vi "Complete Call.vi"(0 "gRPCid":T1, 3 "error in":errorcluster) -> (10 "error out":errorcluster)   [LabVIEW 2019, in "grpc-lvsupport.lvlib"]
uses:
  grpc-lvsupport.lvlib
  grpcId.ctl
  <vilib>/Utility/error.llb/Error Cluster From Error Code.vi
  <resource>/libgrpc_labview.dll
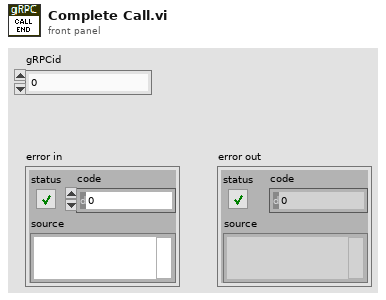
[diagram p1: front panel]
types:
  T1 = typedef "grpc-lvsupport.lvlib/grpcId.ctl" = u64
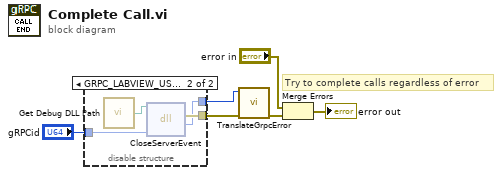
[diagram p0: block diagram]
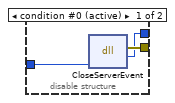
[diagram p2: hidden frame]
diagram:
  # "Try to complete calls regardless of error"
  n1 = disable-structure shown="GRPC_LABVIEW_USE_DEBUG_DLL==True&&RUN_TIME_ENGINE==False" {
    disable-tunnel: [w9 w13] -> w6
    disable-tunnel: "gRPCid" -> [w8 w12]
    disable-tunnel: [w7 w10] -> w3
    frame condition #0 (active) {
      n2 = dll-call lib="C:/Program Files (x86)/National Instruments/LabVIEW 2024/resource/libgrpc_labview.*" fn="CloseServerEvent"("id"=w8) -> (error out=w9:errorcluster, "return type"=w7:i32)  [unwired: 4 in, 1 out]
    }
    frame condition #1 {
      n3 = call "Get Debug DLL Path.vi"() -> ("DLL Path"=w11:path)
      n4 = dll-call lib="?" fn="CloseServerEvent"(path in=w11, "id"=w12) -> (error out=w13:errorcluster, "return type"=w10:i32)  [unwired: 3 in, 1 out]
    }
  }
  n5 = call "TranslateGrpcError.vi"("error in"=w6, "Error Code"=w3) -> ("error out"=w4:errorcluster)  [unwired: 9 in]
  n6 = Merge Errors("error in", w4) -> (→"error out":errorcluster)
